vi "配置向导_串口参数.vi"() -> ()   [LabVIEW 2015]
uses:
  <vilib>/Utility/config.llb/Read Key (String).vi
  <vilib>/Utility/config.llb/Read Key (U32).vi
  <vilib>/Utility/config.llb/NI_LVConfig.lvlib
panel:
  out "err out":errorcluster[](array[cluster])
  in  "error in (no error)":errorcluster caption="错误输入（无错误）"
  in  "输入ini文件地址":path=path "F:/Project/GPRS测试/GPRS测试上位机/GPATS.ini"
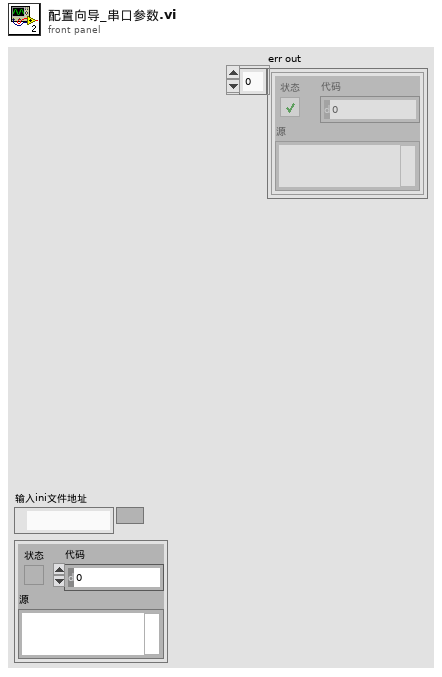
[diagram p1: front panel]
types:
  T1 = typedef "NI_LVConfig.lvlib/Config Data RefNum.ctl" = refnum<k1>
  T2 = enum16{"Left Button", "Center Button", "Right Button", "Window Close"}
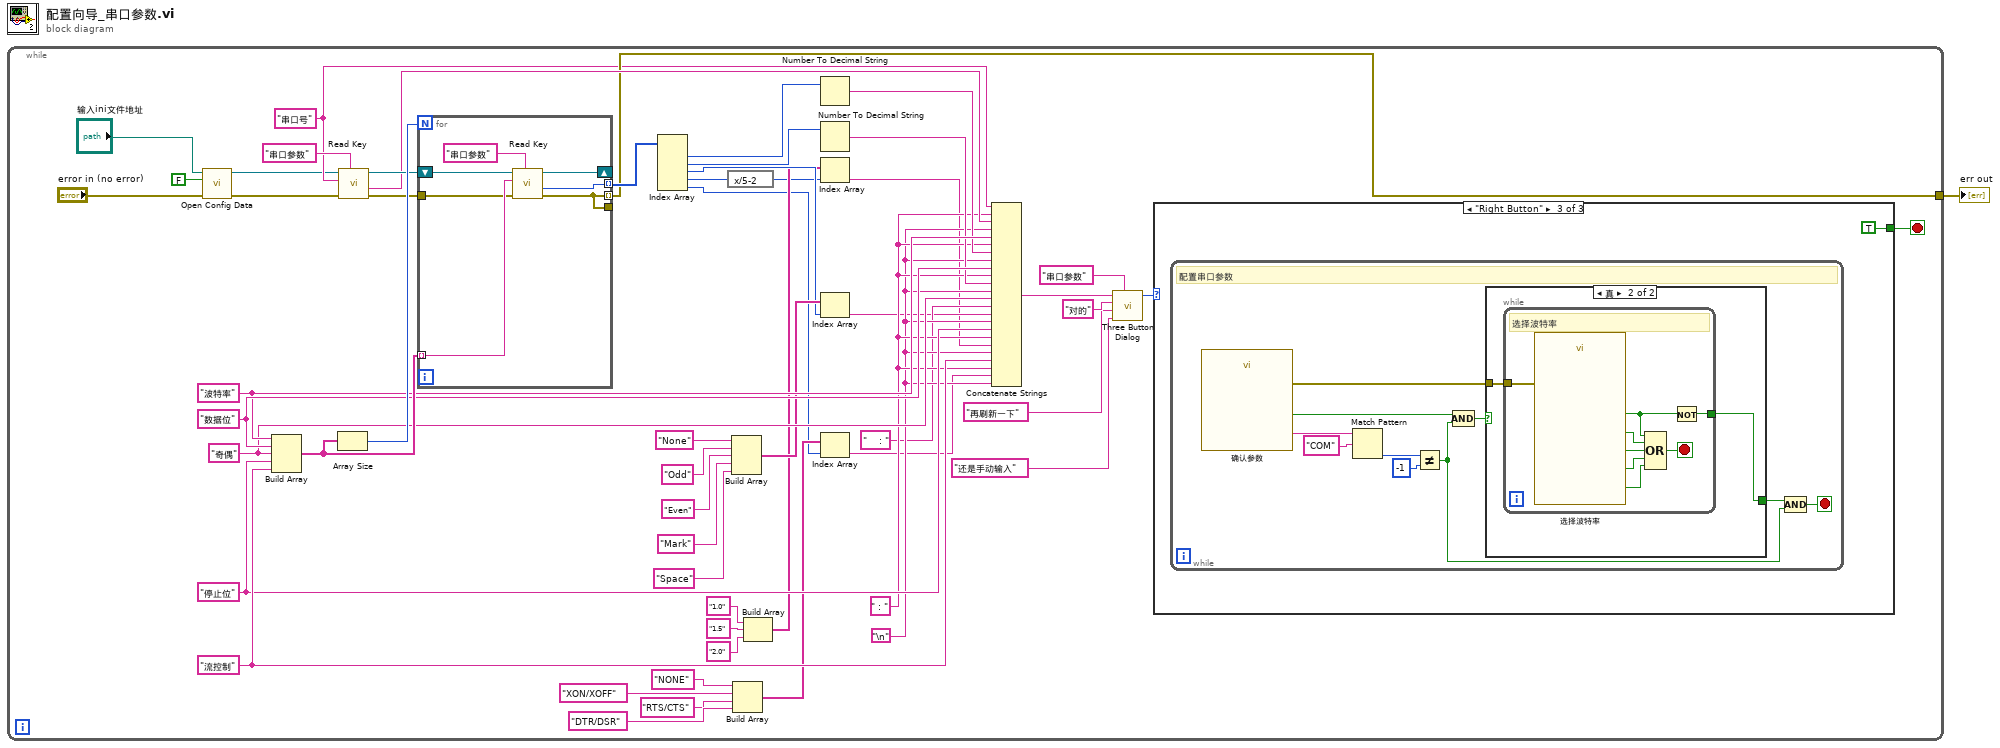
[diagram p0: block diagram]
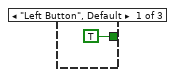
[diagram p2: hidden frame]
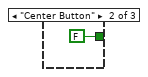
[diagram p3: hidden frame]
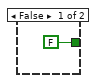
[diagram p4: hidden frame]
diagram:
  n1 = while {
    tunnel: [w40] -> w1
    stop <- w50 stop-if-true
    w31 = " : " ("字符串")
    w30 = "\n"
    w41 = "流控制" ("key")
    w33 = "停止位" ("key")
    w32 = "奇偶" ("key")
    w42 = "数据位" ("key")
    w38 = "波特率" ("key")
    w39 = "串口号" ("key")
    n2 = call <vilib>:"Open Config Data.vi"("error in (no error)"="error in (no error)", "create file if necessary (T)"=FALSE, "configuration file path"="输入ini文件地址") -> ("error out"=w16:errorcluster, "refnum"=w17:T1)  [unwired: 6 in, 1 out]
    n3 = Build Array(w38, w42, w32, w33, w41) -> (w47:string[])
    n4 = Array Size(array=w47) -> (size(s)=w48:i32)
    n5 = call-poly <vilib>:"Read Key.vi"("section"="串口参数" ("key"), "error in (no error)"=w16, "key"=w39, "refnum"=w17) -> ("error out"=w46:errorcluster, "value"=w43:string, "refnum out"=w44:T1)  [unwired: 4 in, 1 out]
    n6 = for {
      N: w48 -> [_]
      tunnel: w47 -> [w62] mode=indexing
      tunnel: [w60] -> w45 mode=indexing
      shift-right: [w59] -> _
      shift-left: w44 -> [w61]
      tunnel: w46 -> [w58]
      tunnel: [w57] -> _
      tunnel: [w57] -> w40 mode=indexing
      n7 = call-poly <vilib>:"Read Key.vi"("section"="串口参数" ("key"), "error in (no error)"=w58, "key"=w62, "refnum"=w61) -> ("error out"=w57:errorcluster, "value"=w60:u32, "refnum out"=w59:T1)  [unwired: 4 in, 1 out]
    }
    n8 = Index Array(array=w45) -> (element #1=w37:u32, element #2=w35:u32, element #3=w22:u32, element #4=w10:u32, element #5=w5:u32)  [unwired: 5 in]
    n9 = expression code="x/5-2"(w10) -> (w11:u32)
    n10 = Build Array("None" ("Left Button Text (\"Yes\")"), "Odd" ("Left Button Text (\"Yes\")"), "Even" ("Left Button Text (\"Yes\")"), "Mark" ("Left Button Text (\"Yes\")"), "Space" ("Left Button Text (\"Yes\")")) -> (w24:string[])
    n11 = Build Array("NONE" ("Left Button Text (\"Yes\")"), "XON/XOFF" ("Left Button Text (\"Yes\")"), "RTS/CTS" ("Left Button Text (\"Yes\")"), "DTR/DSR" ("元素")) -> (w6:string[])
    n12 = Build Array("1.0" ("Left Button Text (\"Yes\")"), "1.5" ("Left Button Text (\"Yes\")"), "2.0" ("Left Button Text (\"Yes\")")) -> (w15:string[])
    n13 = Number To Decimal String(number=w37) -> (decimal integer string=w36:string)  [unwired: 1 in]
    n14 = Number To Decimal String(number=w35) -> (decimal integer string=w34:string)  [unwired: 1 in]
    n15 = Index Array(array=w15, index=w11) -> (element=w9:string)
    n16 = Index Array(array=w24, index=w22) -> (element=w21:string)
    n17 = Index Array(array=w6, index=w5) -> (element=w4:string)
    n18 = Concatenate Strings(w39, w31, w43, w30, w38, w31, w36, w30, w42, w31, w34, w30, w32, "    : " ("字符串"), w21, w30, w33, w31, w9, w30, w41, w31, w4, w30) -> (w56:string)
    n19 = call <vilib>:"Three Button Dialog.vi"("Window Title (\"\")"="串口参数" ("Window Title (\"\")"), "Right Button Text (\"Cancel\")"="还是手动输入" ("Right Button Text (\"Cancel\")"), "Center Button Text (\"No\")"="再刷新一下" ("Center Button Text (\"No\")"), "Left Button Text (\"Yes\")"="对的" ("Left Button Text (\"Yes\")"), "message"=w56) -> ("Which Button?"=w51:T2)  [unwired: 6 in]
    n20 = case shown="\"Right Button\"" w51 {
      tunnel: [TRUE FALSE TRUE] -> w50
      frame "Left Button", Default {
      }
      frame "Center Button" {
      }
      frame "Right Button" {
        n21 = while {
          stop <- w72 stop-if-true
          # "配置串口参数"
          n22 = call "确认参数"() -> ("串口号"=w71:string, "下一步"=w75:bool, "error out"=w76:errorcluster)  [unwired: 17 in]
          n23 = Match Pattern(string=w71, regular expression="COM" ("正则表达式")) -> (offset past match=w69:i32)  [unwired: 1 in, 3 out]
          n24 = Not Equal?(x=w69, y=-1) -> (x != y?=w67:bool)
          n25 = Compound Arithmetic op=AND ("复合运算")(w75, w67) -> (w74:bool)
          n26 = case shown="真" w74 {
            tunnel: w76 -> [_ w79]
            tunnel: [FALSE w78] -> w73
            frame False {
            }
            frame True {
              n27 = while {
                tunnel: w79 -> [w87]
                tunnel: [w81] -> w78
                stop <- w82 stop-if-true
                # "选择波特率"
                n28 = call "选择波特率"("error in (no error)"=w87) -> ("1200"=w83:bool, "4800"=w84:bool, "9600"=w85:bool, "19200"=w86:bool, "上一步"=w80:bool)  [unwired: 13 in, 1 out]
                n29 = Compound Arithmetic op=OR ("复合运算")(w80, w86, w85, w84, w83) -> (w82:bool)
                n30 = Not(x=w80) -> (.not. x?=w81:bool)
              }
            }
          }
          n31 = Compound Arithmetic op=AND ("复合运算")(w73, w67) -> (w72:bool)
        }
      }
    }
  }
  "err out" <- w1
